vi "Osciloskop_main.vi"() -> ()   [LabVIEW 2019]
uses:
  <vilib>/DAQmx/read.llb/DAQmx Read (Analog 1D Wfm NChan NSamp).vi
  <vilib>/measure/mamon.llb/Trigger Detection for 1 Channel.vi
  <vilib>/express/express analysis/Spectral/Block/exnSpectralBlock spectral measurements RMS poly.vi
  <vilib>/express/express analysis/Spectral/Block/exnSpectralBlock spectral measurements RMS array WFM.vi
  <vilib>/DAQmx/create/channels.llb/DAQmx Create Channel (AI-Voltage-Basic).vi
  <vilib>/DAQmx/configure/timing.llb/DAQmx Timing (Sample Clock).vi
  <vilib>/DAQmx/miscellaneous.llb/DAQmx Fill In Error Info.vi
  <vilib>/express/express analysis/Spectral/XNode/ExpressSpectralMeasurementsBlockNode.xnode
  Agilent 33XXX Series/Agilent 33XXX Series.lvlib
  <vilib>/measure/NI_MAPro.lvlib
panel:
  in  "?":T1(tab)
  in  "OFFSET UNITS 0":string(combo)="mV"
  in  "Trigger Enable":bool
  in  "OFFSET 0":dbl
  in  "Channel0_en":bool
  in  "Channel1_en":bool
  in  "Auto adjust":bool
  in  "Cursor1":bool
  out "Waveform Graph":waveform(dbl)[](graph)
  in  "Cursor0":bool
  out "Channel0 Measurements":string
  out "Cursor 0":string
  out "Cursor 1":string
  in  "?":bool
  in  "S/DIV 1":dbl(knob)=0.001 caption="S/DIV" scale=0.001..1.0
  in  "V/DIV 1":dbl(knob)=0.001 caption="V/DIV" scale=0.001..100.0
  out "disp_S/div_1":string
  out "disp_V/div_1":string
  in  "V/DIV 0":dbl(knob)=0.001 scale=0.001..100.0
  in  "S/DIV 0":dbl(knob)=0.001 scale=0.001..1.0
  out "disp_V/div_2":string
  out "disp_S/div_2":string
  in  "TIME OFFSET 1":i32(slide)=1000000 scale=100000.0..1000000.0
  out "Channel1 Measurements":string
  in  "[ESC]":bool
  in  "TIME OFFSET 0":i32(slide)=1000000 scale=100000.0..1000000.0
  in  "OFFSET 1":dbl
  out "Delta Ch0":string
  in  "Trigger slope":u16=1
  in  "Level":dbl format="%.2p"
  in  "OFFSET UNITS 1":string(combo)="mV"
  out "FFT_graph":cluster{"f0":dbl, "df":dbl, "magnitude":dbl[]}[](graph)
  in  "Send settings":bool
  in  "Serial Configuration":T2={"Baud Rate"=9600, "Parity"=0, "Data Bits"=8, "Flow Control"=4} {"Flow Control" items=["None", "XON/XOFF", "RTS/CTS", "XON/XOFF & RTS/CTS", "DTR/DSR", "XON/XOFF & DTR/DSR"]; "Data Bits" items=["7"=7, "8"=8]; "Parity" items=["None", "Odd", "Even", "Mark", "Space"]; "Baud Rate" items=["300"=300, "600"=600, "1200"=1200, "2400"=2400, "4800"=4800, "9600"=9600, "19200"=19200]}
  in  "VISA resource name":refnum<visa-resource-name>
  in  "Amplitude (1 Vpp)":dbl=1.0
  in  "DC Offset (0.00 V)":dbl
  in  "Waveform Function (1: Sine)":u16(ring)=1 items=["DC", "Sine", "Square", "Triangle", "Ramp", "Pulse", "Noise", "Sinc", "Negative Ramp", "Exponential Rise", "Exponential Fall", "Cardiac"]
  in  "Frequency (1000 Hz)":dbl=1000.0
  in  "Physical channels":tag
  in  "SYSTEM SETTINGS":T3={"Sampling frequency [Hz]"=100000.0, "Number of samples"=100000, "Data Buffer size"=1000000, "Sample mode"=10123} {"Sample mode" items=["Finite Samples"=10178, "Continuous Samples"=10123, "Hardware Timed Single Point"=12522]}
  # "DAQ Settings"
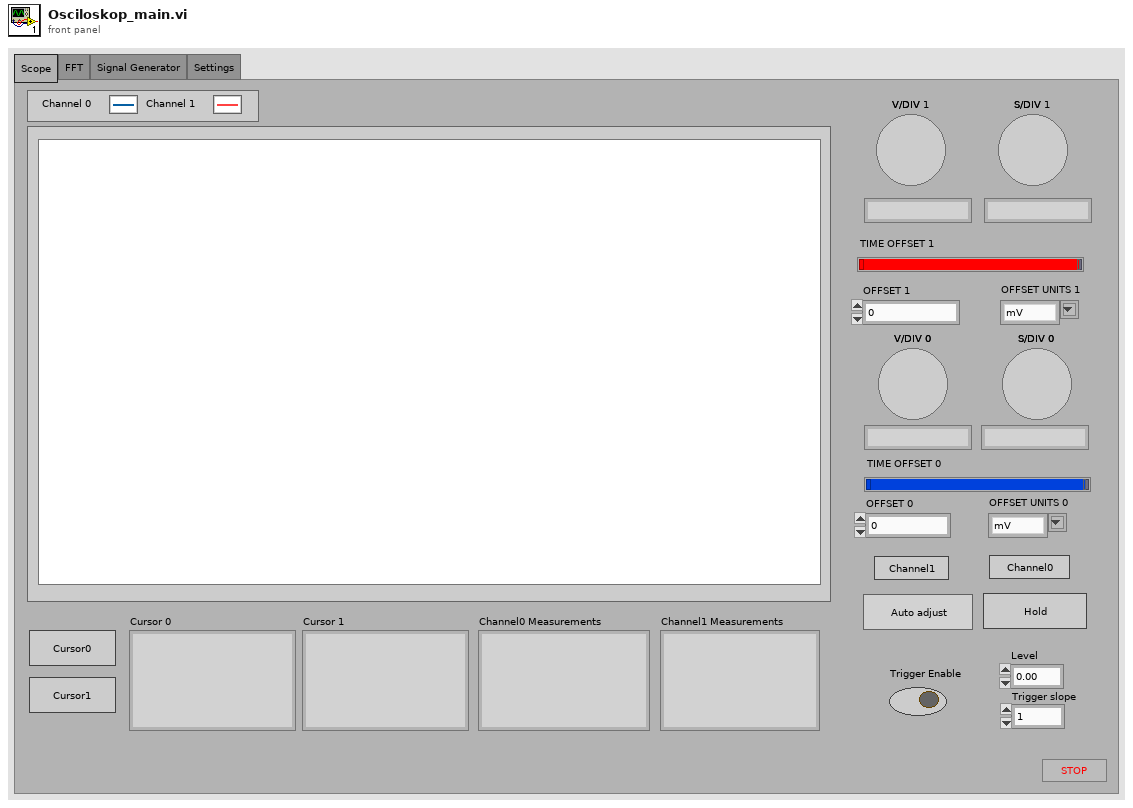
[diagram p1: front panel]
types:
  T1 = enum32{"Scope", "FFT", "Signal Generator", "Settings"}
  T2 = cluster{"Baud Rate":u32, "Parity":u16, "Data Bits":u16, "Flow Control":u16}
  T3 = cluster{"Sampling frequency [Hz]":dbl, "Number of samples":i32, "Data Buffer size":i32, "Sample mode":i32}
  T4 = cluster{"Channel0_en":bool, "Channel1_en":bool, "Auto adjust ":bool, "Cursor0":bool, "Cursor1":bool, "S/DIV":dbl, "V/DIV":dbl, "S/DIV 1":dbl, "V/DIV 1":dbl}
  T5 = cluster{"TIME OFFSET 1":i32, "OFFSET UNIT 0":string, "TIME OFFSET 0":i32, "OFFSET UNIT 1\n":string, "OFFSET 0":dbl, "OFFSET 1":dbl}
  T6 = cluster{"averaging mode":u16, "weighting mode":u16, "number of averages":u32}
  T7 = cluster{"dB On (F)":bool, "unwrap phase (F)":bool, "convert to degree (F)":bool}
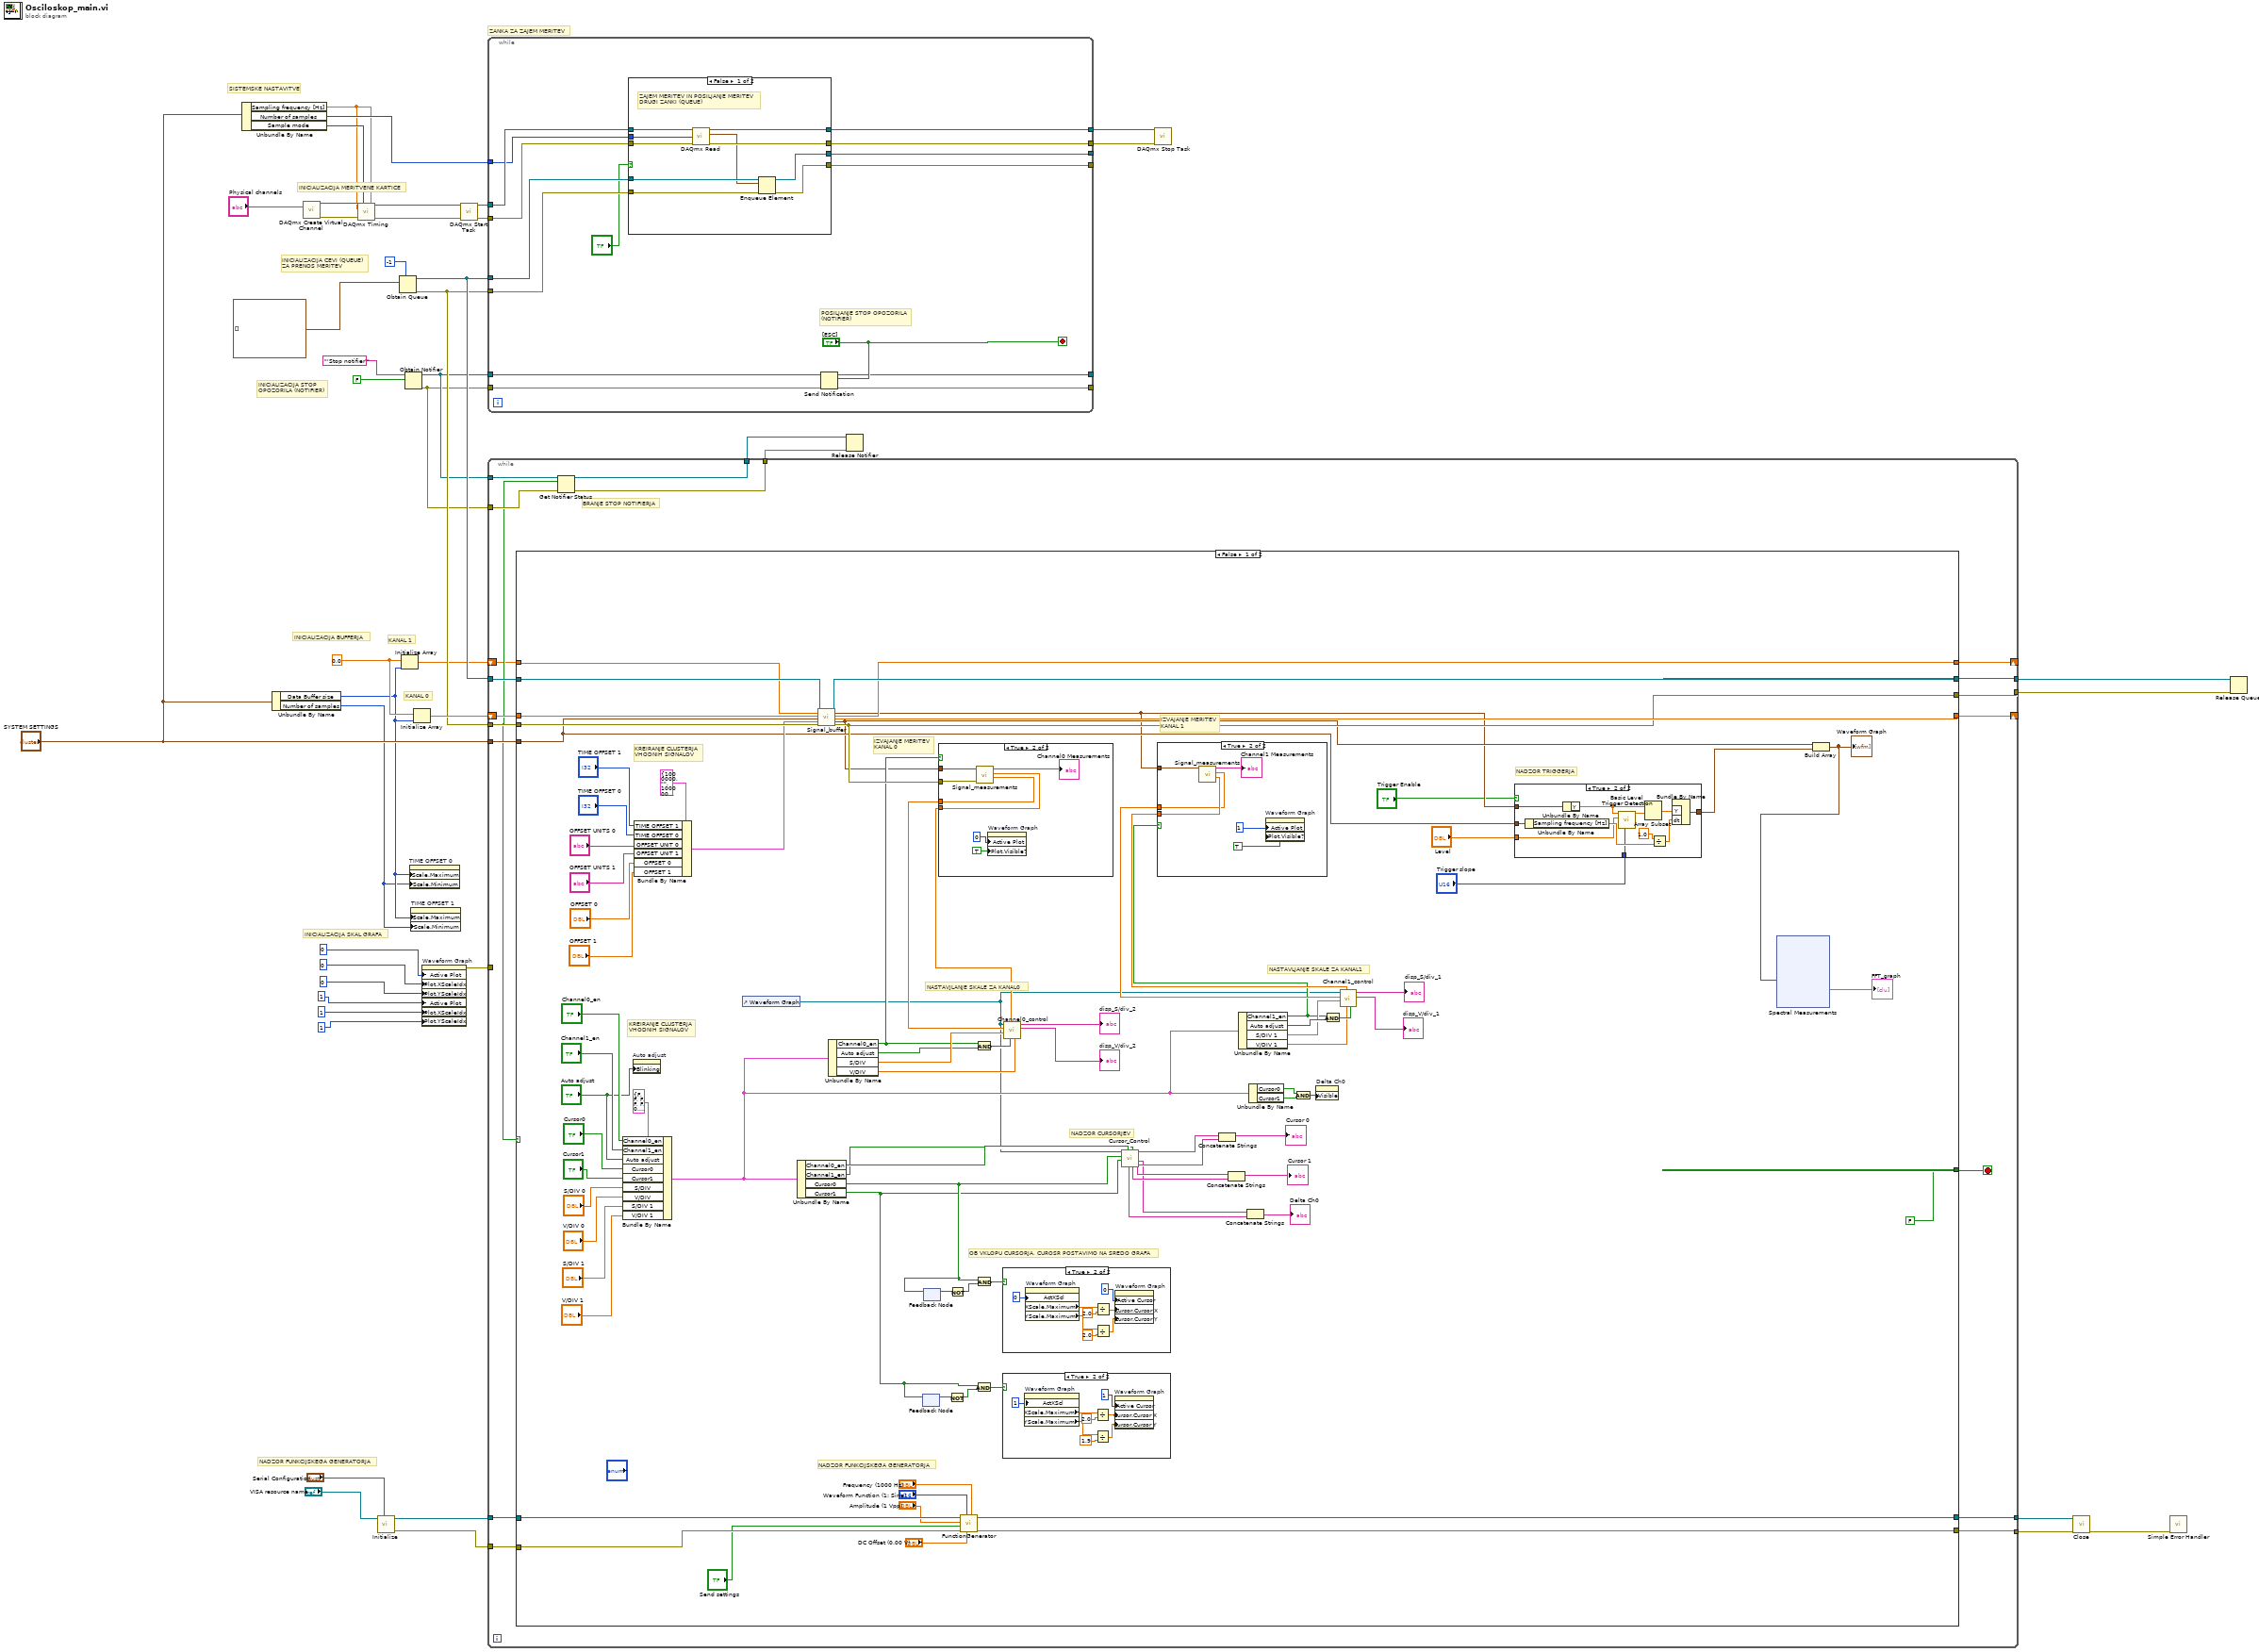
[diagram p0: block diagram]
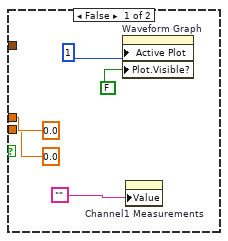
[diagram p6: hidden frame]
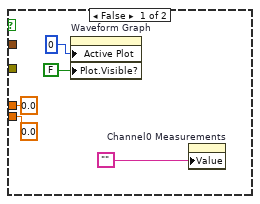
[diagram p7: hidden frame]
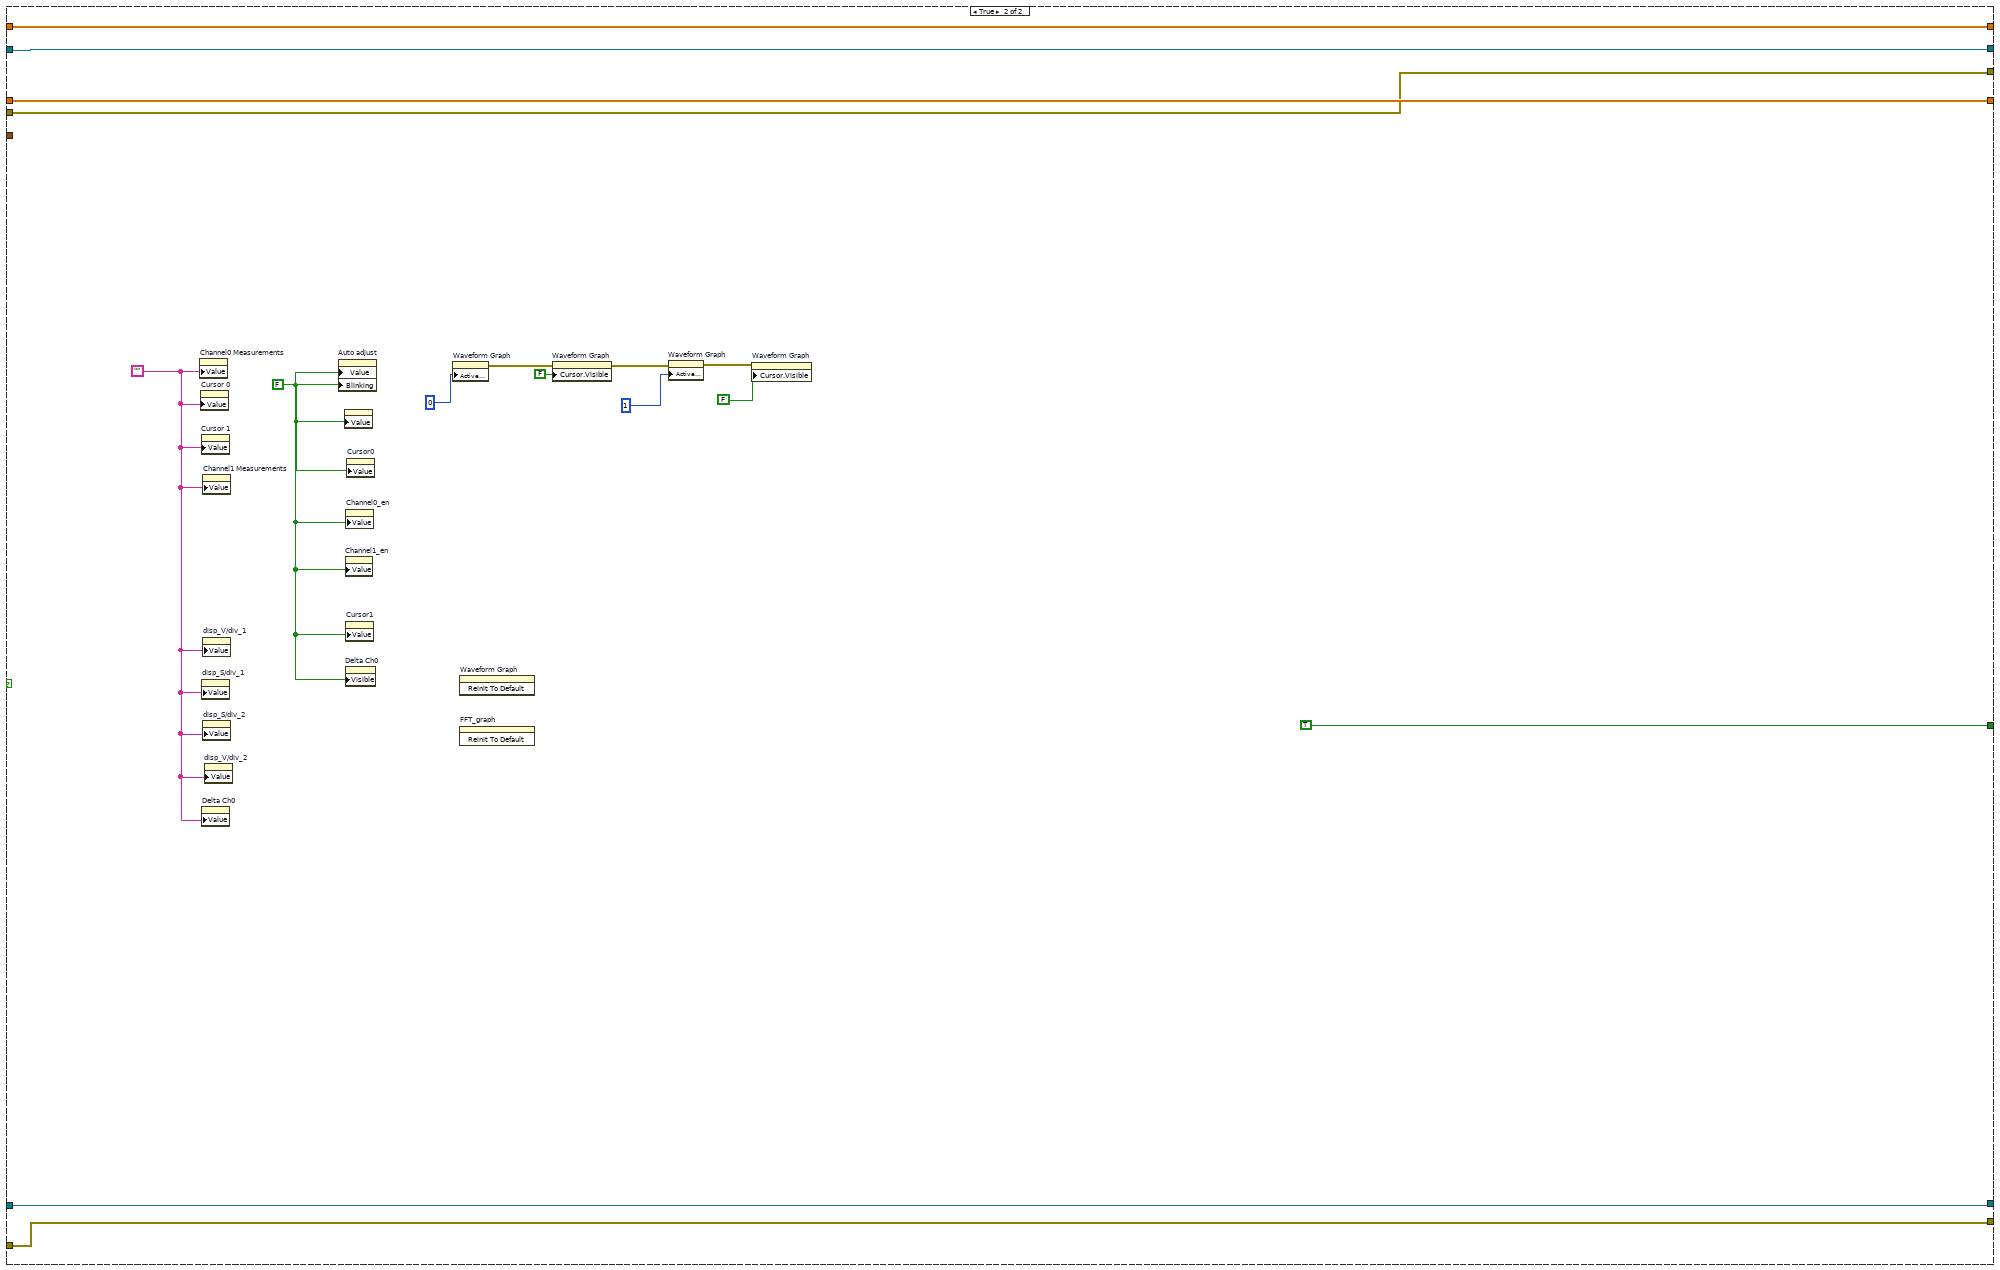
[diagram p8: hidden frame]
diagram:
  w21 = 0.0 ("element")
  # "INICIALIZACIJA SKAL GRAFA"
  # "KANAL 0"
  # "KANAL 1"
  # "INICIALIZACIJA BUFFERJA"
  # "SISTEMSKE NASTAVITVE"
  # "INICIALIZACIJA STOP\nOPOZORILA (NOTIFIER)"
  # "INICIALIZACIJA CEVI (QUEUE)\nZA PRENOS MERITEV"
  # "NADZOR FUNKCIJSKEGA GENERATORJA"
  # "INICIALIZACIJA MERITVENE KARTICE"
  # "ZANKA ZA ZAJEM MERITEV"
  n1 = Unbundle By Name("SYSTEM SETTINGS") -> ("Sampling frequency [Hz]"=w23:dbl, "Number of samples"=w24:i32, "Sample mode"=w33:i32)
  n2 = Unbundle By Name("SYSTEM SETTINGS") -> ("Data Buffer size"=w12:i32, "Number of samples"=w11:i32)
  n3 = call-poly <vilib>:"DAQmx Create Virtual Channel.vi"("physical channels"="Physical channels") -> ("task out"=w43:refnum<k21>, "error out"=w42:errorcluster)  [unwired: 13 in]
  n4 = call-poly <vilib>:"DAQmx Timing.vi"("task/channels in"=w43, "sample mode"=w33, "samples per channel"=w23, "rate"=w23, "error in"=w42) -> ("task out"=w10:refnum<k21>, "error out"=w9:errorcluster)  [unwired: 9 in]
  n5 = call "Initialize.vi"("Serial Configuration"="Serial Configuration", "VISA resource name"="VISA resource name") -> ("error out"=w7:errorcluster, "VISA resource name out"=w8:refnum<visa-resource-name>)  [unwired: 8 in]
  n6 = Obtain Queue(max queue size (-1, unlimited)=-1, element data type=waveform(dbl)[] []) -> (queue out=w36:refnum<queue>, error out=w35:errorcluster)  [unwired: 3 in, 1 out]
  n7 = Initialize Array(w21, w12) -> (w20:dbl[])
  n8 = Obtain Notifier(name (unnamed)="'Stop notifier'", notification data type=FALSE) -> (notifier out=w30:refnum<notifier>, error out=w29:errorcluster)  [unwired: 2 in, 1 out]
  n9 = property on="TIME OFFSET 0" class="Slide (strict)"("Scale.Maximum"=w12, "Scale.Minimum"=w11) -> ()  [unwired: 2 in, 2 out]
  n10 = property on="TIME OFFSET 1" class="Slide (strict)"("Scale.Maximum"=w12, "Scale.Minimum"=w11) -> ()  [unwired: 2 in, 2 out]
  n11 = Initialize Array(w21, w12) -> (w44:dbl[])
  n12 = property on="Waveform Graph" class="WFGraph (strict)"("Active Plot"=u32 0, "Plot.XScaleIdx"=u32 0 ("Plot.X Scale Index"), "Plot.YScaleIdx"=u32 0 ("Plot.Y Scale Index"), "Active Plot"=u32 1, "Plot.XScaleIdx"=u32 1 ("Plot.X Scale Index"), "Plot.YScaleIdx"=u32 1 ("Plot.Y Scale Index")) -> (error out=w17:errorcluster)  [unwired: 2 in, 1 out]
  n13 = call <vilib>:"DAQmx Start Task.vi"("task/channels in"=w10, "error in"=w9) -> ("task out"=w41:refnum<k21>, "error out"=w40:errorcluster)  [unwired: 12 in]
  n14 = while {
    shift-right: [w60] -> _
    shift-left: w44 -> [w61]
    tunnel: w36 -> [w63]
    tunnel: w35 -> [w62]
    tunnel: "SYSTEM SETTINGS" -> [w59]
    tunnel: w30 -> [w56]
    tunnel: w29 -> [w55]
    tunnel: [w58] -> w28
    tunnel: [w57] -> w27
    tunnel: [w54] -> w26
    tunnel: [w53] -> w25
    shift-right: [w49] -> _
    shift-left: w20 -> [w50]
    tunnel: w17 -> [_]
    tunnel: w8 -> [w48]
    tunnel: w7 -> [w47]
    tunnel: [w46] -> w6
    tunnel: [w45] -> w5
    stop <- w51 stop-if-true
    # "BRANJE STOP NOTIFIERJA"
    n15 = Get Notifier Status(notifier=w56, error in (no error)=w55) -> (notifier out=w54:refnum<notifier>, current notification=w52:bool, error out=w53:errorcluster)  [unwired: 2 out]
    n16 = case shown="False" w52 {
      tunnel: w63 -> [w148 w226]
      tunnel: w62 -> [w147 w225]
      tunnel: w61 -> [w146 w227]
      tunnel: [w134 w227] -> w60
      tunnel: w59 -> [w90 _]
      tunnel: [w145 w226] -> w58
      tunnel: [w130 w225] -> w57
      tunnel: [FALSE TRUE] -> w51
      tunnel: w50 -> [w143 w216]
      tunnel: [w135 w216] -> w49
      tunnel: w48 -> [w139 w214]
      tunnel: w47 -> [w138 w213]
      tunnel: [w136 w214] -> w46
      tunnel: [w137 w213] -> w45
      frame False {
        # "NADZOR TRIGGERJA"
        # "NASTAVLJANJE SKALE ZA KANAL1"
        # "KREIRANJE CLUSTERJA\nVHODNIH SIGNALOV"
        # "KREIRANJE CLUSTERJA \nVHODNIH SIGNALOV"
        # "NADZOR FUNKCIJSKEGA GENERATORJA"
        # "OB VKLOPU CURSORJA, CUROSR POSTAVIMO NA SREDO GRAFA"
        # "NADZOR CURSORJEV"
        # "NASTAVJLANJE SKALE ZA KANAL0"
        # "IZVAJANJE MERITEV\nKANAL 1"
        # "IZVAJANJE MERITEV\nKANAL 0"
        n17 = Bundle By Name(cluster=T4 {"Channel0_en"=FALSE, "Channel1_en"=FALSE, "Auto adjust "=FALSE, "Cursor0"=FALSE, "Cursor1"=FALSE, "S/DIV"=0.0, "V/DIV"=0.0, "S/DIV 1"=0.0, "V/DIV 1"=0.0}, "Channel0_en"="Channel0_en", "Channel1_en"="Channel1_en", "Auto adjust"="Auto adjust", "Cursor0"="Cursor0", "Cursor1"="Cursor1", "S/DIV"="S/DIV 0", "V/DIV"="V/DIV 0", "S/DIV 1"="S/DIV 1", "V/DIV 1"="V/DIV 1") -> (w92:T4)
        n18 = property on="Auto adjust" class="Bool (strict)"("Blinking"="Auto adjust") -> ()  [unwired: 2 in, 2 out]
        n19 = Bundle By Name(cluster=T5 {"TIME OFFSET 1"=1000000, "OFFSET UNIT 0"="", "TIME OFFSET 0"=1000000, "OFFSET UNIT 1\n"="", "OFFSET 0"=0.0, "OFFSET 1"=0.0} ("Input controls (cluster)"), "TIME OFFSET 1"="TIME OFFSET 1", "TIME OFFSET 0"="TIME OFFSET 0", "OFFSET UNIT 0"="OFFSET UNITS 0", "OFFSET UNIT 1"="OFFSET UNITS 1", "OFFSET 0"="OFFSET 0", "OFFSET 1"="OFFSET 1") -> (w121:T5)
        n20 = control-ref of="Waveform Graph"() -> (w91:refnum<vi>)
        n21 = Unbundle By Name(w92) -> ("Channel0_en"=w105:bool, "Channel1_en"=w104:bool, "Cursor0"=w80:bool, "Cursor1"=w76:bool)
        n22 = call "Signal_buffer.vi"("Queue in"=w148, "Bufer1 IN"=w143, "Buffer0 IN"=w146, "SYSTEM SETTINGS"=w90, "Input controls (cluster)"=w121, "error in (no error)"=w147) -> ("Queue out"=w145:refnum<queue>, "Waveform 1"=w88:waveform(dbl), "Buffer1 OUT"=w135:dbl[], "Buffer0 OUT"=w134:dbl[], "Waveform 0"=w89:waveform(dbl), "error out"=w130:errorcluster)  [unwired: 8 in]
        n23 = Unbundle By Name(w92) -> ("Channel0_en"=w96:bool, "Auto adjust"=w101:bool, "S/DIV"=w103:dbl, "V/DIV"=w102:dbl)
        n24 = feedback #1() -> (w79:bool)  [unwired: 1 in]
        n25 = feedback-in #1(w76) -> ()
        n26 = feedback-in #2(w80) -> ()
        n27 = feedback #2() -> (w81:bool)  [unwired: 1 in]
        n28 = case shown="True" w96 {
          tunnel: w130 -> [_ w208]
          tunnel: w89 -> [_ w207]
          tunnel: [0.0 ("Measured frequency") w206] -> w133
          tunnel: [0.0 ("Measured amplitude") w205] -> w132
          frame False {
            n29 = property on="Waveform Graph" class="WFGraph (strict)"("Active Plot"=u32 0, "Plot.Visible?"=FALSE ("Plot.Visible")) -> ()  [unwired: 2 in, 2 out]
            n30 = property on="Channel0 Measurements" class="Str"("Value"="") -> ()  [unwired: 2 in, 2 out]
          }
          frame True {
            n31 = call "Signal_measurements.vi"("error in (no error)"=w208, "Input waveform"=w207) -> ("Measured frequency"=w206:dbl, "Measured amplitude"=w205:dbl, "String"=→"Channel0 Measurements":string)  [unwired: 6 in, 1 out]
            n32 = property on="Waveform Graph" class="WFGraph (strict)"("Active Plot"=u32 0, "Plot.Visible?"=TRUE ("Plot.Visible")) -> ()  [unwired: 2 in, 2 out]
          }
        }
        n33 = Not(x=w79) -> (.not. x?=w78:bool)
        n34 = Not(x=w81) -> (.not. x?=w82:bool)
        n35 = call "FunctionGenerator.vi"("Frequency (1000 Hz)"="Frequency (1000 Hz)", "DC Offset (0.00 V)"="DC Offset (0.00 V)", "Waveform Function (1: Sine)"="Waveform Function (1: Sine)", "error in (no error)"=w138, "Send settings"="Send settings", "Amplitude (1 Vpp)"="Amplitude (1 Vpp)", "VISA Refnum in"=w139) -> ("error out"=w137:errorcluster, "VISA Refnum out"=w136:refnum<visa-resource-name>)  [unwired: 3 in]
        n36 = And(x=w76, y=w78) -> (x .and. y?=w77:bool)
        n37 = And(x=w96, y=w101) -> (x .and. y?=w131:bool)
        n38 = And(x=w80, y=w82) -> (x .and. y?=w83:bool)
        n39 = case shown="True" w77 {
          frame False {
          }
          frame True {
            n40 = property on="Waveform Graph" class="WFGraph (strict)"("ActXScl"=1 ("Active X Scale")) -> ("XScale.Maximum"=w167:dbl, "YScale.Maximum"=w161:dbl)  [unwired: 2 in, 2 out]
            n41 = Divide(x=w167, y=2.0) -> (x/y=w168:dbl)
            n42 = Divide(x=w161, y=1.9) -> (x/y=w162:dbl)
            n43 = property on="Waveform Graph" class="WFGraph (strict)"("Active Cursor"=u32 1, "Cursor.Cursor X"=w168, "Cursor.Cursor Y"=w162) -> ()  [unwired: 2 in, 2 out]
          }
        }
        n44 = case shown="True" w83 {
          frame False {
          }
          frame True {
            n45 = property on="Waveform Graph" class="WFGraph (strict)"("ActXScl"=0 ("Active X Scale")) -> ("XScale.Maximum"=w175:dbl, "YScale.Maximum"=w169:dbl)  [unwired: 2 in, 2 out]
            n46 = Divide(x=w175, y=2.0) -> (x/y=w176:dbl)
            n47 = Divide(x=w169, y=2.0) -> (x/y=w170:dbl)
            n48 = property on="Waveform Graph" class="WFGraph (strict)"("Active Cursor"=u32 0, "Cursor.Cursor X"=w176, "Cursor.Cursor Y"=w170) -> ()  [unwired: 2 in, 2 out]
          }
        }
        n49 = call "Channel0_control.vi"("V/DIV in"=w102, "Boolean"=w131, "Measured amplitude"=w132, "S/DIV in"=w103, "Measured frequency"=w133, "WaveformGraph in"=w91) -> ("V/DIV out"=→"disp_V/div_2":string, "S/DIV out"=→"disp_S/div_2":string)  [unwired: 4 in]
        n50 = call "Cursor_Control.vi"("Channel 1 EN"=w104, "Channel 0 EN"=w105, "Cursor1 ON"=w76, "Curso0 ON"=w80, "WaveformGraph in"=w91) -> ("Cursor0_Scale1_disp"=w118:string, "Delta Ch0"=w84:string, "Cursor1_Scale0_disp"=w116:string, "Cursor0_Scale0_disp"=w119:string, "Cursor1_Scale1_disp"=w115:string, "Delta Ch1"=w85:string)  [unwired: 1 in]
        n51 = Concatenate Strings(w119, w118) -> (→"Cursor 0":string)
        n52 = Concatenate Strings(w116, w115) -> (→"Cursor 1":string)
        n53 = Unbundle By Name(w92) -> ("Channel1_en"=w95:bool, "Auto adjust"=w100:bool, "S/DIV 1"=w98:dbl, "V/DIV 1"=w99:dbl)
        n54 = case shown="True" w95 {
          tunnel: w88 -> [_ w196]
          tunnel: [0.0 ("Measured amplitude") w195] -> w129
          tunnel: [0.0 ("Measured frequency") w194] -> w128
          frame False {
            n55 = property on="Waveform Graph" class="WFGraph (strict)"("Active Plot"=u32 1, "Plot.Visible?"=FALSE ("Plot.Visible")) -> ()  [unwired: 2 in, 2 out]
            n56 = property on="Channel1 Measurements" class="Str"("Value"="") -> ()  [unwired: 2 in, 2 out]
          }
          frame True {
            n57 = call "Signal_measurements.vi"("Input waveform"=w196) -> ("Measured frequency"=w195:dbl, "Measured amplitude"=w194:dbl, "String"=→"Channel1 Measurements":string)  [unwired: 7 in, 1 out]
            n58 = property on="Waveform Graph" class="WFGraph (strict)"("Active Plot"=u32 1, "Plot.Visible?"=TRUE ("Plot.Visible")) -> ()  [unwired: 2 in, 2 out]
          }
        }
        n59 = Concatenate Strings(w84, w85) -> (→"Delta Ch0":string)
        n60 = Unbundle By Name(w92) -> ("Cursor0"=w94:bool, "Cursor1"=w93:bool)
        n61 = And(x=w94, y=w93) -> (x .and. y?=w140:bool)
        n62 = property on="Delta Ch0" class="Str"("Visible"=w140) -> ()  [unwired: 2 in, 2 out]
        n63 = And(x=w95, y=w100) -> (x .and. y?=w127:bool)
        n64 = call "Channel1_control.vi"("Auto adjust ON"=w127, "V/DIV 1"=w99, "Measured frequency"=w129, "S/DIV 1"=w98, "Measured amplitude"=w128, "WaveformGraph in"=w91) -> ("V/DIV out"=→"disp_V/div_1":string, "S/DIV out"=→"disp_S/div_1":string)  [unwired: 4 in]
        n65 = case shown="True" "Trigger Enable" {
          tunnel: w90 -> [_ w188]
          tunnel: w88 -> [w177 w184]
          tunnel: [w177 w183] -> w87
          tunnel: "Level" -> [_ w179]
          tunnel: "Trigger slope" -> [_ w178]
          frame False {
          }
          frame True {
            n66 = Unbundle By Name(w188) -> ("Sampling frequency [Hz]"=w185:dbl)
            n67 = Unbundle By Name(w184) -> ("Y"=w182:dbl[])
            n68 = call-poly <vilib>:"Basic Level Trigger Detection.vi"("signal in"=w182, "level"=w179, "trigger slope"=w178) -> ("trigger location"=w180:dbl)  [unwired: 10 in, 2 out]
            n69 = Array Subset(array=w182, index=w180) -> (w181:dbl[])  [unwired: 1 in]
            n70 = Divide(x=1.0, y=w185) -> (x/y=w186:dbl)
            n71 = Bundle By Name("Y"=w181, "dt"=w186) -> (w183:waveform(dbl))  [unwired: 1 in]
          }
        }
        n72 = Build Array(w89, w87) -> (w74:waveform(dbl)[])
        "Waveform Graph" <- w74
        n73 = xnode "Spectral Measurements"("Signals"=w74) -> ("FFT - (RMS)"=→"FFT_graph":cluster{"f0":dbl, "df":dbl, "magnitude":dbl[]}[])  [unwired: 1 in, 2 out]
      }
      frame True {
        w212 = FALSE ("Blinking")
        w215 = ""
        n74 = property on="Channel0 Measurements" class="Str"("Value"=w215) -> ()  [unwired: 2 in, 2 out]
        n75 = property on="Cursor 0" class="Str"("Value"=w215) -> ()  [unwired: 2 in, 2 out]
        n76 = property on="Cursor 1" class="Str"("Value"=w215) -> ()  [unwired: 2 in, 2 out]
        n77 = property on="disp_S/div_1" class="Str"("Value"=w215) -> ()  [unwired: 2 in, 2 out]
        n78 = property on="Delta Ch0" class="Str"("Value"=w215) -> ()  [unwired: 2 in, 2 out]
        n79 = property on="Channel1 Measurements" class="Str"("Value"=w215) -> ()  [unwired: 2 in, 2 out]
        n80 = property on="disp_V/div_1" class="Str"("Value"=w215) -> ()  [unwired: 2 in, 2 out]
        n81 = property on="disp_S/div_2" class="Str"("Value"=w215) -> ()  [unwired: 2 in, 2 out]
        n82 = property on="disp_V/div_2" class="Str"("Value"=w215) -> ()  [unwired: 2 in, 2 out]
        n83 = property on="Auto adjust" class="Bool (strict)"("Value"=w212, "Blinking"=w212) -> ()  [unwired: 2 in, 2 out]
        n84 = property class="Bool (strict)"("Value"=w212) -> ()  [unwired: 2 in, 2 out]
        n85 = property on="Channel1_en" class="Bool (strict)"("Value"=w212) -> ()  [unwired: 2 in, 2 out]
        n86 = property on="Delta Ch0" class="Str"("Visible"=w212) -> ()  [unwired: 2 in, 2 out]
        n87 = property on="Channel0_en" class="Bool (strict)"("Value"=w212) -> ()  [unwired: 2 in, 2 out]
        n88 = property on="Cursor1" class="Bool (strict)"("Value"=w212) -> ()  [unwired: 2 in, 2 out]
        n89 = property on="Cursor0" class="Bool (strict)"("Value"=w212) -> ()  [unwired: 2 in, 2 out]
        n90 = property on="Waveform Graph" class="WFGraph (strict)"("Active Cursor"=u32 0) -> (error out=w223:errorcluster)  [unwired: 2 in, 1 out]
        n91 = invoke on="Waveform Graph" class="WFGraph (strict)" method="Reinit To Default"() -> ()  [unwired: 3 in, 3 out]
        n92 = invoke on="FFT_graph" class="WFGraph (strict)" method="Reinit To Default"() -> ()  [unwired: 3 in, 3 out]
        n93 = property on="Waveform Graph" class="WFGraph (strict)"(error in=w223, "Cursor.Visible"=FALSE) -> (error out=w220:errorcluster)  [unwired: 1 in, 1 out]
        n94 = property on="Waveform Graph" class="WFGraph (strict)"(error in=w220, "Active Cursor"=u32 1) -> (error out=w221:errorcluster)  [unwired: 1 in, 1 out]
        n95 = property on="Waveform Graph" class="WFGraph (strict)"(error in=w221, "Cursor.Visible"=FALSE) -> ()  [unwired: 1 in, 2 out]
      }
    }
  }
  n96 = while {
    tunnel: w36 -> [w242]
    tunnel: [w240] -> _
    tunnel: w35 -> [w241]
    tunnel: [w239] -> _
    tunnel: w40 -> [w237]
    tunnel: [w235] -> w38
    tunnel: w41 -> [w238]
    tunnel: [w236] -> w39
    tunnel: w24 -> [w234]
    tunnel: w30 -> [w231]
    tunnel: [w230] -> _
    tunnel: [w229] -> _
    tunnel: w29 -> [w228]
    stop <- "[ESC]" stop-if-true
    # "POSILJANJE STOP OPOZORILA\n(NOTIFIER)"
    n97 = case shown="False" "?" {
      tunnel: w242 -> [w252 w254]
      tunnel: w241 -> [w251 w253]
      tunnel: [w250 w254] -> w240
      tunnel: [w249 w253] -> w239
      tunnel: w238 -> [w248 w256]
      tunnel: w237 -> [w247 w255]
      tunnel: [w246 w256] -> w236
      tunnel: [w245 w255] -> w235
      tunnel: w234 -> [w244 _]
      frame False {
        # "ZAJEM MERITEV IN POSILJANJE MERITEV \nDRUGI ZANKI (QUEUE)"
        n98 = call-poly <vilib>:"DAQmx Read.vi"("task/channels in"=w248, "number of samples per channel"=w244, "error in"=w247) -> ("task out"=w246:refnum<k21>, "data"=w243:waveform(dbl)[], "error out"=w245:errorcluster)  [unwired: 10 in]
        n99 = Enqueue Element(queue=w252, element=w243, error in (no error)=w251) -> (queue out=w250:refnum<queue>, error out=w249:errorcluster)  [unwired: 1 in, 1 out]
      }
      frame True {
      }
    }
    n100 = Send Notification(notification="[ESC]", notifier=w231, error in (no error)=w228) -> (notifier out=w230:refnum<notifier>, error out=w229:errorcluster)
  }
  n101 = Release Notifier(notifier=w26, error in (no error)=w25) -> ()  [unwired: 1 in, 3 out]
  n102 = call <vilib>:"DAQmx Stop Task.vi"("task/channels in"=w39, "error in"=w38) -> ()  [unwired: 12 in, 2 out]
  n103 = call "Close.vi"("error in (no error)"=w5, "VISA resource name"=w6) -> ("error out"=w2:errorcluster)  [unwired: 9 in]
  n104 = call <vilib>:"Simple Error Handler.vi"("error in (no error)"=w2) -> ()  [unwired: 4 in, 5 out]
  n105 = Release Queue(queue=w28, error in (no error)=w27) -> ()  [unwired: 1 in, 3 out]
